vi "REPORT_AUDIT_add_value_to_results.vi"(0 "records_input":string[][](array[string]), 3 "results":string[][](array[string]), 5 "operation_statuses_input":T1[](array[typedef])) -> (4 "records_output":string[][](array[string]), 6 "operation_statuses_ouptup":T1[](array[typedef]), 8 "additionally_row":i32)   [LabVIEW 2020]
uses:
  GEAR/typedef/REPORT_GEAR_statuses.ctl
  <userlib>/_OpenG.lib/array/array.llb/Filter 1D Array with Scalar (String)__ogtk.vi
  _misc/AULocalize/SubVIs/Get Localized Phrase Compact Interface 1D.vi
  _misc/AULocalize/SubVIs/Get Localized Phrase Compact Interface 2D.vi
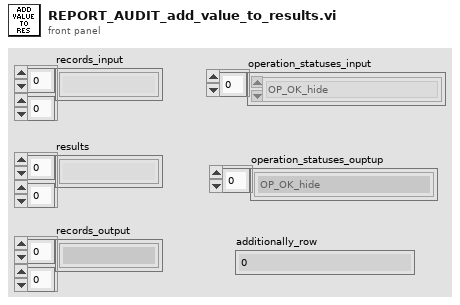
[diagram p1: front panel]
types:
  T1 = typedef "REPORT_GEAR_statuses.ctl" = enum16{"OP_OK_hide", "OP_OK_show", "OP_NOK_hide", "OP_NOK_show", "OP_interrupted_hide", "OP_interrupted_show", "OP_in_operation_hide", "OP_in_operation_show", "OP_unexpected_hide", "OP_unexpected_show", "RE_REAL_OK", "RE_REAL_NOK", "RE_STRING", "RE_sub_header", "RE_no_data", "RE_unexpected", "BA_sub_header", "BA_data", "BA_no_data"}
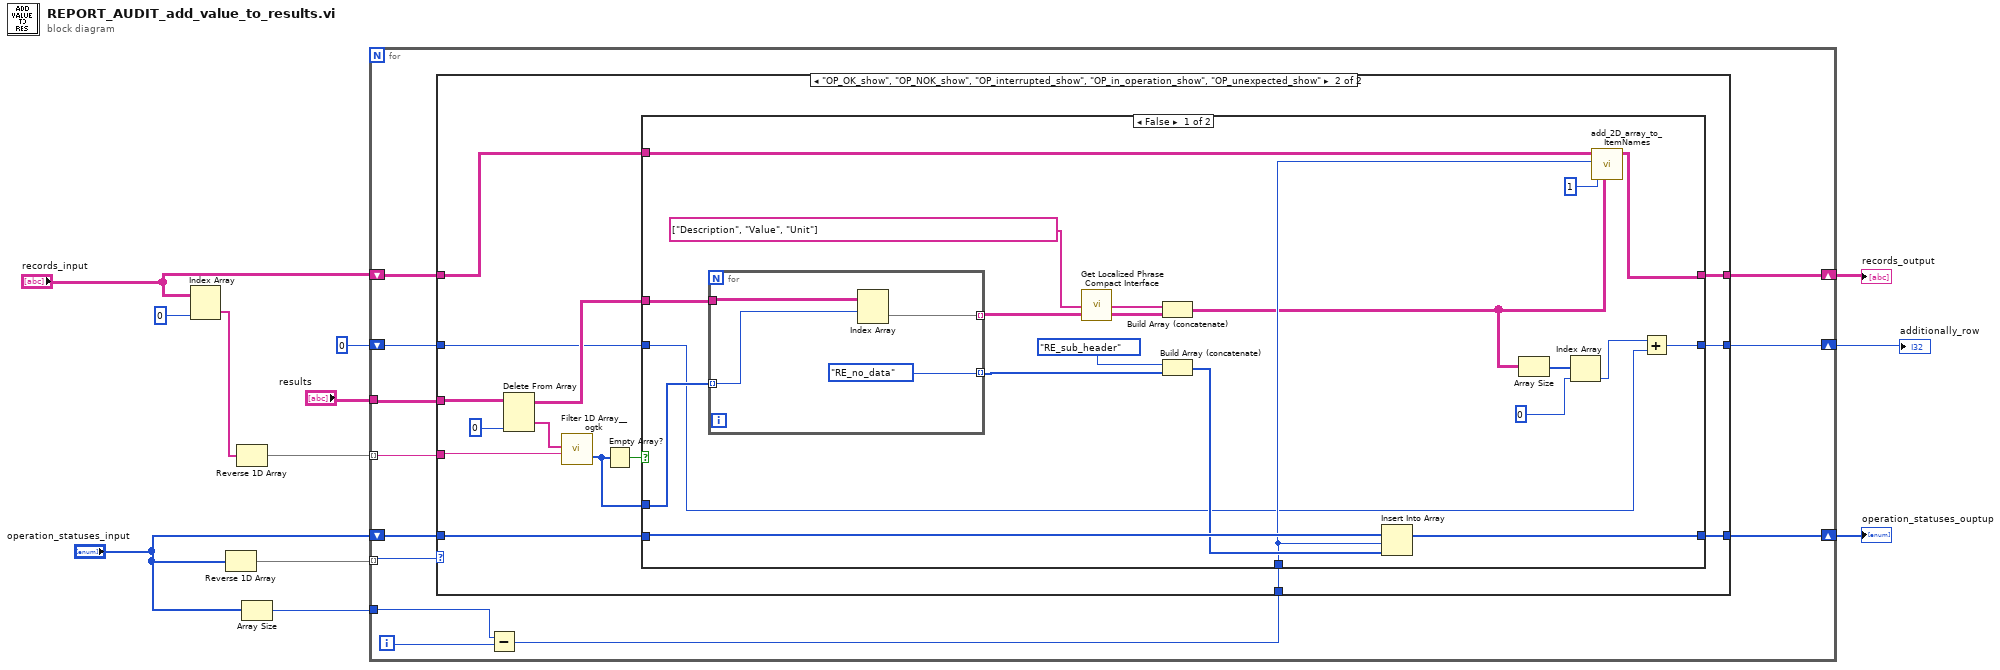
[diagram p0: block diagram]
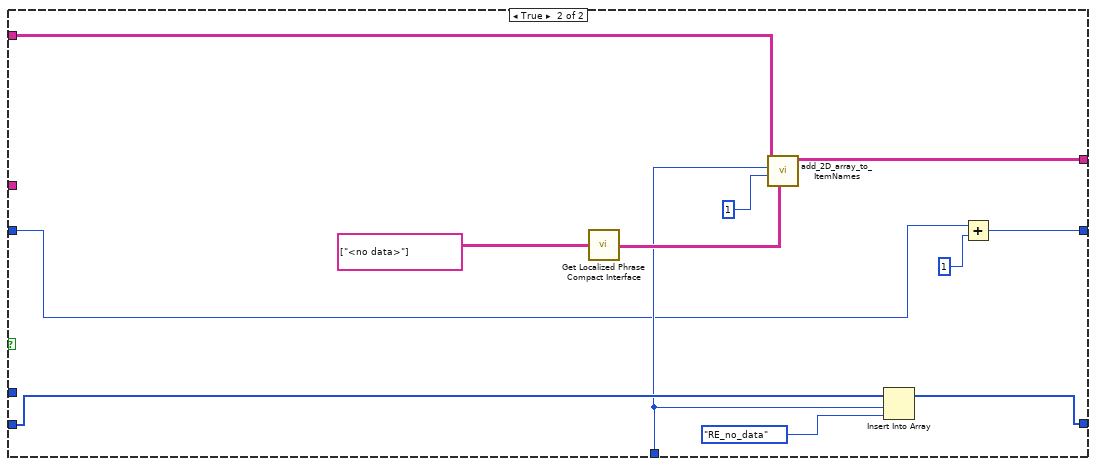
[diagram p3: hidden frame]
diagram:
  n1 = Index Array(array="records_input", index (col)=0 ("disabled index (col)")) -> (element=w7:string[])  [unwired: 1 in]
  n2 = Reverse 1D Array(array="operation_statuses_input") -> (reversed array=w5:T1[])
  n3 = Reverse 1D Array(array=w7) -> (reversed array=w6:string[])
  n4 = Array Size(array="operation_statuses_input") -> (size(s)=w3:i32)
  n5 = for {
    tunnel: w5 -> [w24] mode=indexing
    tunnel: "results" -> [w23]
    shift-right: [w21] -> w11
    shift-left: "records_input" -> [w22]
    shift-right: [w19] -> w10
    shift-left: "operation_statuses_input" -> [w20]
    tunnel: w6 -> [w18] mode=indexing
    tunnel: w3 -> [w17]
    shift-right: [w13] -> w1
    shift-left: 0 -> [w14]
    i -> [w16]
    n6 = Subtract(x=w17, y=w16) -> (x-y=w15:i32)
    n7 = case shown="\"OP_OK_show\", \"OP_NOK_show\", \"OP_interrupted_show\", \"OP_in_operation_show\", \"OP_unexpected_show\"" w24 {
      tunnel: w23 -> [_ w40]
      tunnel: w22 -> [w27 w35]
      tunnel: w18 -> [_ w30]
      tunnel: [w27 w34] -> w21
      tunnel: w20 -> [w26 w33]
      tunnel: w15 -> [_ w32]
      tunnel: [w26 w31] -> w19
      tunnel: w14 -> [w25 w29]
      tunnel: [w25 w28] -> w13
      frame Default {
      }
      frame "OP_OK_show", "OP_NOK_show", "OP_interrupted_show", "OP_in_operation_show", "OP_unexpected_show" {
        n8 = Delete From Array(array=w40, index (col)=0 ("disabled index (col)")) -> (deleted portion=w39:string[], array with subset deleted=w36:string[][])  [unwired: 2 in]
        n9 = call-poly <userlib>:"Filter 1D Array__ogtk.vi"("items to filter"=w30, "array"=w39) -> ("filtered item indices"=w37:i32[])  [unwired: 4 in, 1 out]
        n10 = Empty Array?(array=w37) -> (empty?=w38:bool)
        n11 = case shown="False" w38 {
          tunnel: w36 -> [w52 _]
          tunnel: [w59 w74] -> w34
          tunnel: w37 -> [w53 _]
          tunnel: w35 -> [w61 w70]
          tunnel: w33 -> [w58 w72]
          tunnel: w32 -> [w48 w69]
          tunnel: [w49 w71] -> w31
          tunnel: w29 -> [w43 w68]
          tunnel: [w42 w66] -> w28
          frame False {
            n12 = for {
              tunnel: w52 -> [w65]
              tunnel: [w64] -> w57 mode=indexing
              tunnel: w53 -> [w63] mode=indexing
              tunnel: [REPORT_GEAR_statuses."RE_no_data" ("REPORT_GEAR_statuses")] -> w50 mode=indexing
              n13 = Index Array(array=w65, index (row)=w63) -> (element=w64:string[])  [unwired: 1 in]
            }
            n14 = call-poly "Get Localized Phrase Compact Interface.vi"("Key"=string[] ["Description", "Value", "Unit"]) -> ("Translated Phrase"=w55:string[])
            n15 = Build Array (concatenate)(w55, w57) -> (w47:string[][])
            n16 = Build Array (concatenate)(REPORT_GEAR_statuses."RE_sub_header" ("REPORT_GEAR_statuses"), w50) -> (w51:T1[])
            n17 = Insert Into Array(array=w58, index=w48, new element=w51) -> (w49:T1[])
            n18 = Array Size(array=w47) -> (size(s)=w46:i32[])
            n19 = Index Array(array=w46, index=0) -> (element=w44:i32)
            n20 = call "add_2D_array_to_ItemNames.vi"("2D_array"=w47, "column"=1, "row"=w48, "ItemNames_in"=w61) -> ("ItemNames_out"=w59:string[][])  [unwired: 7 in]
            n21 = Add(x=w44, y=w43) -> (x+y=w42:i32)
          }
          frame True {
            n22 = call-poly "Get Localized Phrase Compact Interface.vi"("Key"=string[][] [["<no data>"]] ("2D_array")) -> ("Translated Phrase"=w75:string[][])
            n23 = call "add_2D_array_to_ItemNames.vi"("2D_array"=w75, "column"=1, "row"=w69, "ItemNames_in"=w70) -> ("ItemNames_out"=w74:string[][])  [unwired: 7 in]
            n24 = Insert Into Array(array=w72, index=w69, new element=REPORT_GEAR_statuses."RE_no_data" ("new element/subarray")) -> (w71:T1[])
            n25 = Add(x=w68, y=1) -> (x+y=w66:i32)
          }
        }
      }
    }
  }
  "records_output" <- w11
  "operation_statuses_ouptup" <- w10
  "additionally_row" <- w1
